vi "Extra_Analysis_info.vi"(1 "Timescales":dbl[](array[numeric]), 2 "Indicies":i32[](array[numeric]), 3 "Analysis type cluster":T1) -> (0 "Values":string[](array[string]))   [LabVIEW 2010]
uses:
  Controls/Analysis_type_cluster.ctl
  Controls/Analysis_type_Enum.ctl
  Controls/Instrument_Array.ctl
  Controls/Post_Process.ctl
  Globals/Meas_global.vi
  Acquisition/PWA/PWAtasksGLOBAL.vi
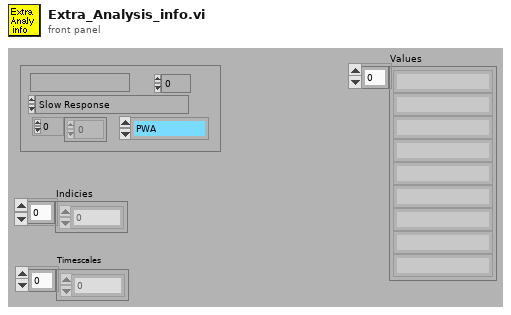
[diagram p1: front panel]
types:
  T1 = typedef "Analysis_type_cluster.ctl" = cluster{"Analysis type":T2, "Indicies":i32[], "Name":string, "Inst Array":T3, "Info index":i32}
  T2 = typedef "Analysis_type_Enum.ctl" = enum16{"Slow Response", "Fast Response", "Weighted Fast Response", "Fast FID", "Weighted Fast FID", "Cross Wire", "Weighted Cross Wire", "Weighted LDA"}
  T3 = typedef "Instrument_Array.ctl" = enum16{"PWA", "LDA", "Analogue"}
  T4 = typedef "Velocity_cluster.ctl" = cluster{"Name":string, "U":dbl, "u^2":dbl, "u^3/(u^2)^(1.5)":dbl, "u^4/(u^2)^2 -3":dbl, "% u'/U":dbl, "Mean % Err":dbl, "u^4":dbl}
  T5 = typedef "Analysis_info_cluster.ctl" = cluster{"Colour":u32, "Inst type":T6, "Inst name":string, "Symbol":string, "Code name":string, "Extra Info":string, "Inst Array":T3, "Index":i32, "Voltage Index":i32, "Extra Titles":string[], "Extra Values":string[]}
  T6 = typedef "Inst_type.ctl" = enum16{"Propeller anemometer", "Raw voltage", "Pressure Transducer", "Pitot-static tube", "Preston tube", "Hot wire", "Cross wire 1", "Cross wire 2", "Generic Linear", "Generic Polynomial", "Generic BackPoly", "Fast FID", "Thermocouple", "Cold wire", "Pulsed Wire", "LDA Vel", "LDA Tran time", "LDA Arr time"}
  T7 = typedef "Post_Process.ctl" = enum16{"Take New Data", "Post Process Raw Data File"}
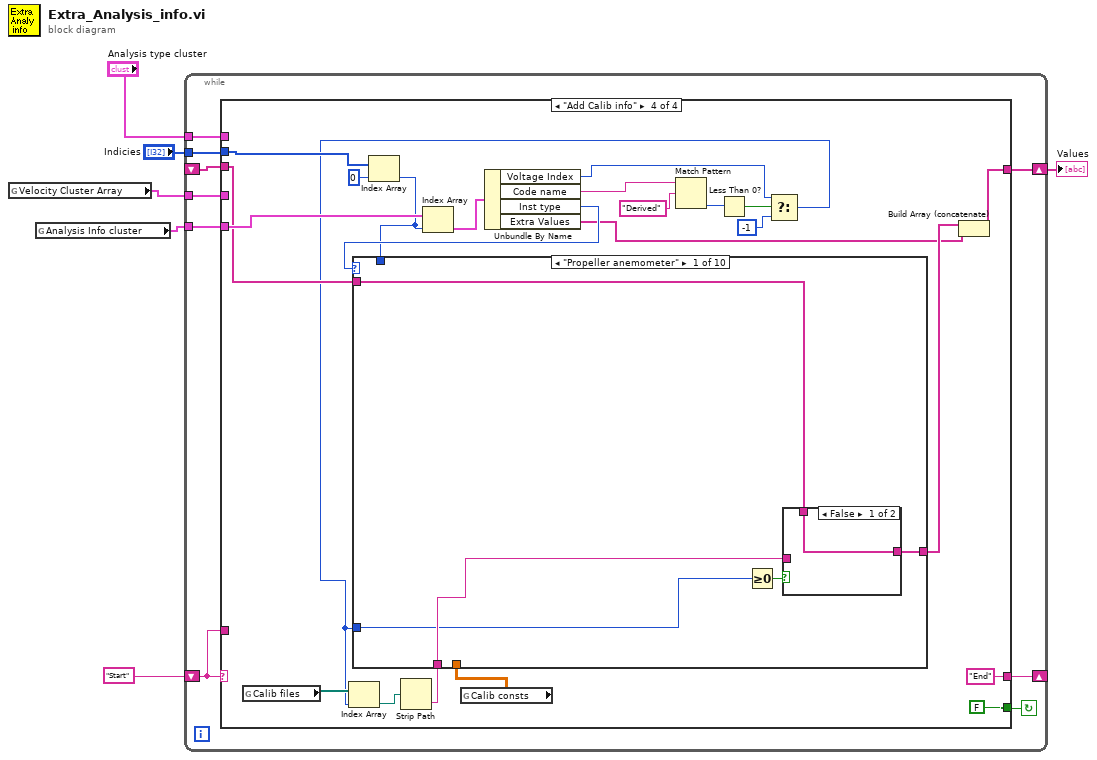
[diagram p0: block diagram]
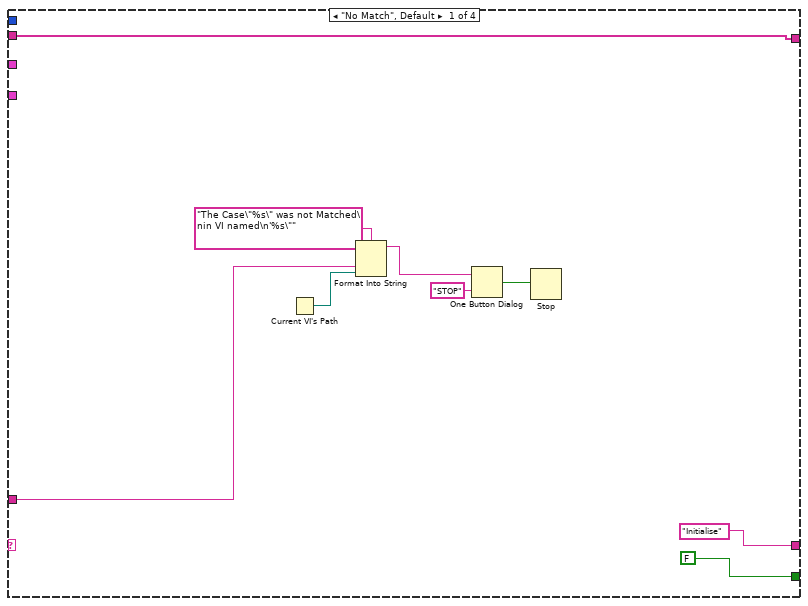
[diagram p2: hidden frame]
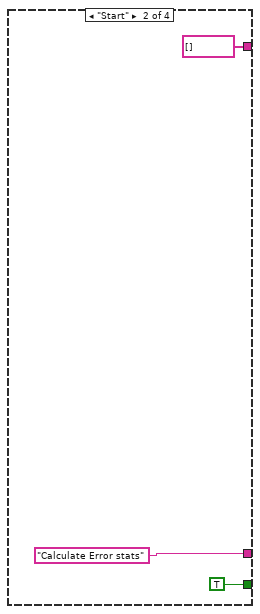
[diagram p3: hidden frame]
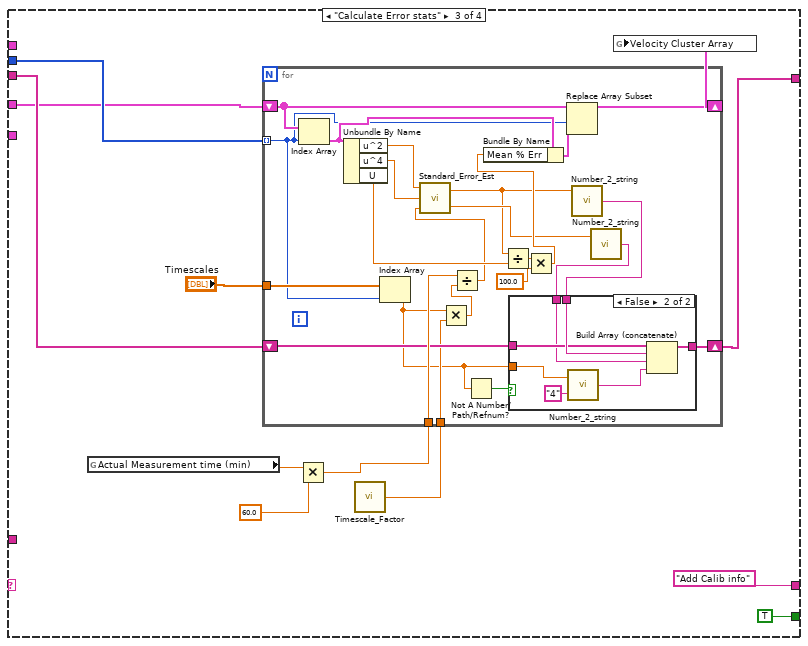
[diagram p4: hidden frame]
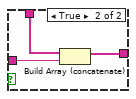
[diagram p6: hidden frame]
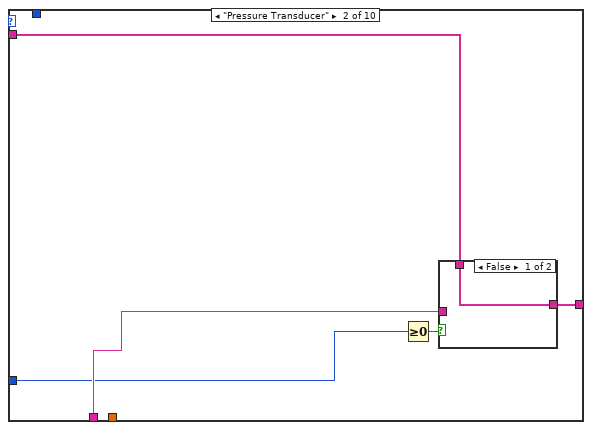
[diagram p7: hidden frame]
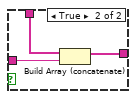
[diagram p8: hidden frame]
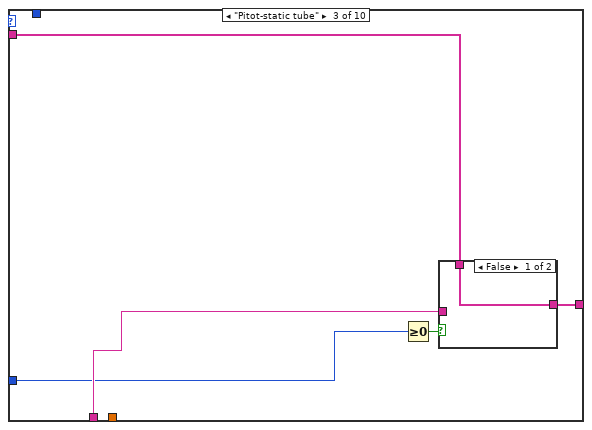
[diagram p9: hidden frame]
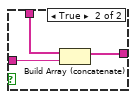
[diagram p10: hidden frame]
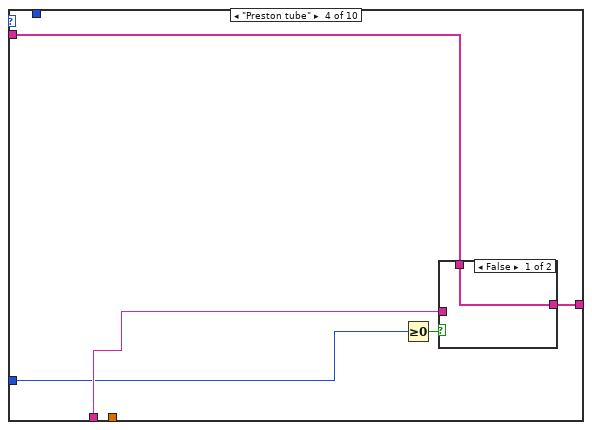
[diagram p11: hidden frame]
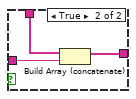
[diagram p12: hidden frame]
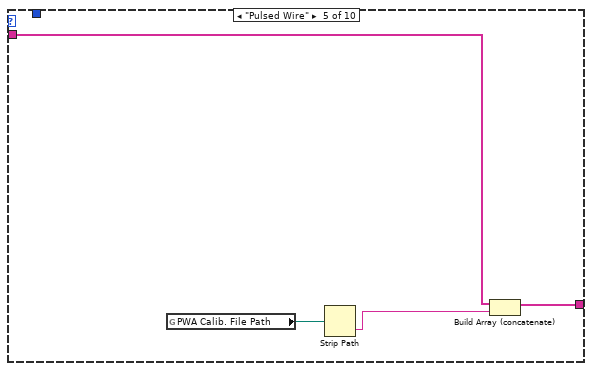
[diagram p13: hidden frame]
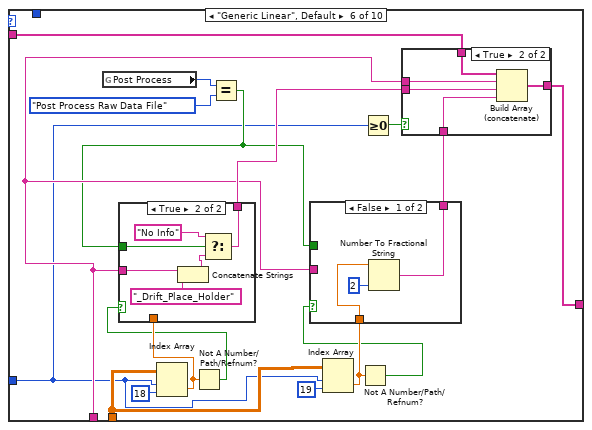
[diagram p14: hidden frame]
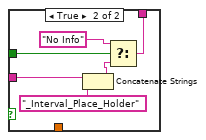
[diagram p16: hidden frame]
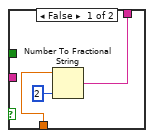
[diagram p17: hidden frame]
diagram:
  n1 = global read "Meas_global.vi" "Velocity Cluster Array"() -> (w1:T4[])
  n2 = global read "Meas_global.vi" "Analysis Info cluster"() -> (w3:T5[])
  n3 = while {
    shift-left: "Start" -> [w13]
    shift-right: [w14] -> _
    tunnel: "Analysis type cluster" -> [w12]
    shift-right: [w10] -> w4
    shift-left: _ -> [w11]
    tunnel: w3 -> [w9]
    tunnel: "Indicies" -> [w8]
    tunnel: w1 -> [w7]
    stop <- w15 continue-if-true
    n4 = case shown="\"Add Calib info\"" w13 {
      tunnel: [FALSE TRUE TRUE FALSE] -> w15
      tunnel: ["Initialise" "Calculate Error stats" "Add Calib info" "End" ("f")] -> w14
      tunnel: w13 -> [w19 _ _ _]
      tunnel: w12 -> [_ _ _ _]
      tunnel: w8 -> [_ _ w35 w82]
      tunnel: w11 -> [w16 _ w37 w90]
      tunnel: [w16 string[] [] w36 w72] -> w10
      tunnel: w9 -> [_ _ _ w93]
      tunnel: w7 -> [_ _ w28 _]
      frame "No Match", Default {
        n5 = Current VI's Path() -> (path=w18:path)
        n6 = Format Into String(format string="The Case\"%s\" was not Matched\nin VI named\n'%s\"" ("Format String"), w19, w18) -> (resulting string=w22:string)  [unwired: 2 in, 1 out]
        n7 = One Button Dialog(message=w22, button name ("OK")="STOP") -> (true=w20:bool)
        n8 = Stop(stop? (T)=w20) -> ()
      }
      frame "Start" {
      }
      frame "Calculate Error stats" {
        n9 = global read "Meas_global.vi" "Actual Measurement time (min)"() -> (w32:dbl)
        n10 = Multiply(x=w32, y=60.0) -> (x*y=w31:dbl)
        n11 = call "Timescale_Factor.vi"() -> ("Factor to scale timescale by"=w33:dbl)
        n12 = for {
          shift-right: [w62] -> w38
          shift-left: w28 -> [w63]
          tunnel: w35 -> [w42] mode=indexing
          tunnel: "Timescales" -> [w55]
          tunnel: w31 -> [w54]
          shift-right: [w51] -> w36
          shift-left: w37 -> [w52]
          tunnel: w33 -> [w50]
          n13 = Index Array(array=w63, index=w42) -> (element=w61:T4)
          n14 = Unbundle By Name(w61) -> ("u^2"=w47:dbl, "u^4"=w46:dbl, "U"=w59:dbl)
          n15 = Index Array(array=w55, index=w42) -> (element=w40:dbl)
          n16 = Multiply(x=w40, y=w50) -> (x*y=w49:dbl)
          n17 = Divide(x=w54, y=w49) -> (x/y=w45:dbl)
          n18 = call "Standard_Error_Est.vi"("N"=w45, "4th order moment u^4"=w46, "2nd order moment u^2"=w47) -> ("Standard error in variance"=w44:dbl, "Standard error in Mean"=w43:dbl)
          n19 = Not A Number/Path/Refnum?(number/path/refnum=w40) -> (NaN/Path/Refnum?=w41:bool)
          n20 = Divide(x=w43, y=w59) -> (x/y=w58:dbl)
          n21 = Multiply(x=w58, y=100.0) -> (x*y=w56:dbl)
          n22 = Bundle By Name(cluster=w61, "Mean % Err"=w56) -> (w60:T4)
          n23 = Replace Array Subset(array=w63, new element=w60, index=w42) -> (w62:T4[])
          n24 = call "Number_2_string.vi"("number"=w43) -> ("String"=w53:string)  [unwired: 1 in]
          n25 = call "Number_2_string.vi"("number"=w44) -> ("String"=w48:string)  [unwired: 1 in]
          n26 = case shown="False" w41 {
            tunnel: w40 -> [_ w70]
            tunnel: w53 -> [_ w69]
            tunnel: w52 -> [w64 w68]
            tunnel: [w64 w67] -> w51
            tunnel: w48 -> [_ w65]
            frame True {
            }
            frame False {
              n27 = call "Number_2_string.vi"("precision"="4", "number"=w70) -> ("String"=w66:string)
              n28 = Build Array (concatenate)(w68, w69, w65, w66) -> (w67:string[])
            }
          }
        }
        n29 = global write "Meas_global.vi" "Velocity Cluster Array"(w38) -> ()
      }
      frame "Add Calib info" {
        n30 = global read "Meas_global.vi" "Calib files"() -> (w89:path[])
        n31 = Index Array(array=w82, index=0 ("Index")) -> (element=w83:i32)
        n32 = Index Array(array=w93, index=w83) -> (element=w92:T5)
        n33 = global read "Meas_global.vi" "Calib consts"() -> (w86:dbl[][])
        n34 = Unbundle By Name(w92) -> ("Voltage Index"=w77:i32, "Code name"=w79:string, "Inst type"=w91:T6, "Extra Values"=w73:string[])
        n35 = Match Pattern(string=w79, regular expression="Derived") -> (offset past match=w80:i32)  [unwired: 4 out]
        n36 = Less Than 0?(x=w80) -> (x < 0?=w78:bool)
        n37 = Select(t=w77, s=w78, f=-1) -> (s? t:f=w75:i32)
        n38 = Index Array(array=w89, index=w75) -> (element=w88:path)
        n39 = Strip Path(path=w88) -> (name=w87:string)  [unwired: 1 out]
        n40 = case shown="\"Propeller anemometer\"" w91 {
          tunnel: [w98 w107 w116 w125 w133 w150 w176 w177 w178 w179] -> w74
          tunnel: w90 -> [w99 w108 w117 w126 w134 w151 w176 w177 w178 w179]
          tunnel: w83 -> [_ _ _ _ _ _ _ _ _ _]
          tunnel: w87 -> [w97 w106 w115 w124 _ w143 _ _ _ _]
          tunnel: w86 -> [_ _ _ _ _ w141 _ _ _ _]
          tunnel: w75 -> [w95 w104 w113 w122 _ w135 _ _ _ _]
          frame "Propeller anemometer" {
            n41 = Greater Or Equal To 0?(x=w95) -> (x >= 0?=w96:bool)
            n42 = case shown="False" w96 {
              tunnel: w99 -> [w100 w103]
              tunnel: [w100 w102] -> w98
              tunnel: w97 -> [_ w101]
              frame False {
              }
              frame True {
                n43 = Build Array (concatenate)(w103, w101) -> (w102:string[])
              }
            }
          }
          frame "Pressure Transducer" {
            n44 = Greater Or Equal To 0?(x=w104) -> (x >= 0?=w105:bool)
            n45 = case shown="False" w105 {
              tunnel: w108 -> [w109 w112]
              tunnel: [w109 w111] -> w107
              tunnel: w106 -> [_ w110]
              frame False {
              }
              frame True {
                n46 = Build Array (concatenate)(w112, w110) -> (w111:string[])
              }
            }
          }
          frame "Pitot-static tube" {
            n47 = Greater Or Equal To 0?(x=w113) -> (x >= 0?=w114:bool)
            n48 = case shown="False" w114 {
              tunnel: w117 -> [w118 w121]
              tunnel: [w118 w120] -> w116
              tunnel: w115 -> [_ w119]
              frame False {
              }
              frame True {
                n49 = Build Array (concatenate)(w121, w119) -> (w120:string[])
              }
            }
          }
          frame "Preston tube" {
            n50 = Greater Or Equal To 0?(x=w122) -> (x >= 0?=w123:bool)
            n51 = case shown="False" w123 {
              tunnel: w126 -> [w127 w130]
              tunnel: [w127 w129] -> w125
              tunnel: w124 -> [_ w128]
              frame False {
              }
              frame True {
                n52 = Build Array (concatenate)(w130, w128) -> (w129:string[])
              }
            }
          }
          frame "Pulsed Wire" {
            n53 = global read "PWAtasksGLOBAL.vi" "PWA Calib. File Path"() -> (w132:path)
            n54 = Strip Path(path=w132) -> (name=w131:string)  [unwired: 1 out]
            n55 = Build Array (concatenate)(w134, w131) -> (w133:string[])
          }
          frame "Generic Linear", Default {
            n56 = global read "Meas_global.vi" "Post Process"() -> (w145:T7)
            n57 = Index Array(array=w141, index (row)=w135, index (col)=18 ("Index")) -> (element=w148:dbl)
            n58 = Not A Number/Path/Refnum?(number/path/refnum=w148) -> (NaN/Path/Refnum?=w147:bool)
            n59 = Equal?(x=w145, y=Post_Process."Post Process Raw Data File" ("Post Process")) -> (x = y?=w137:bool)
            n60 = case shown="True" w147 {
              tunnel: [w167 w172] -> w144
              tunnel: w148 -> [w168 _]
              tunnel: w137 -> [_ w174]
              tunnel: w143 -> [_ w171]
              frame False {
                n61 = Number To Fractional String(number=w168, precision (6)=i16 2) -> (F-format string=w167:string)  [unwired: 2 out]
              }
              frame True {
                n62 = Concatenate Strings(w171, "_Drift_Place_Holder" ("Substring")) -> (w173:string)
                n63 = Select(t="No Info", s=w174, f=w173) -> (s? t:f=w172:string)
              }
            }
            n64 = Index Array(array=w141, index (row)=w135, index (col)=19 ("Index")) -> (element=w140:dbl)
            n65 = Not A Number/Path/Refnum?(number/path/refnum=w140) -> (NaN/Path/Refnum?=w139:bool)
            n66 = case shown="False" w139 {
              tunnel: [w158 w163] -> w138
              tunnel: w140 -> [w159 _]
              tunnel: w137 -> [_ w165]
              tunnel: w143 -> [_ w162]
              frame False {
                n67 = Number To Fractional String(number=w159, precision (6)=i16 2) -> (F-format string=w158:string)  [unwired: 2 out]
              }
              frame True {
                n68 = Concatenate Strings(w162, "_Interval_Place_Holder" ("Substring")) -> (w164:string)
                n69 = Select(t="No Info", s=w165, f=w164) -> (s? t:f=w163:string)
              }
            }
            n70 = Greater Or Equal To 0?(x=w135) -> (x >= 0?=w136:bool)
            n71 = case shown="True" w136 {
              tunnel: w151 -> [w152 w157]
              tunnel: [w152 w156] -> w150
              tunnel: w144 -> [_ w155]
              tunnel: w143 -> [_ w154]
              tunnel: w138 -> [_ w153]
              frame False {
              }
              frame True {
                n72 = Build Array (concatenate)(w157, w154, w155, w153) -> (w156:string[])
              }
            }
          }
          frame "Raw voltage" {
          }
          frame "LDA Vel" {
          }
          frame "LDA Tran time" {
          }
          frame "LDA Arr time" {
          }
        }
        n73 = Build Array (concatenate)(w74, w73) -> (w72:string[])
      }
    }
  }
  "Values" <- w4
